vi "Live_Spectrum.vi"() -> ()   [LabVIEW 2022 SP3]
uses:
  PreferencesControl.ctl
  Mic/Mic_Global.vi
  <vilib>/sound2/lvsound2.llb/Sound Input Read (DBL).vi
panel:
  in  "Mode":enum16{"Single Shot", "Continuous"}(ring)
  out "Hammer FFT":cluster{"x0":dbl, "df":dbl, dbl[]}(graph)
  out "Microphone FFT":cluster{"x0":dbl, "df":dbl, dbl[]}(graph)
  in  "Fire":bool
  out "Hammer":waveform(dbl)(graph)
  out "Microphone":waveform(dbl)(graph)
  out "Settings":T1={"Name of test"="", "Date"=timestamp(0 s since 1904-01-01), "Location"="", "Template"="", "Soundcard"="", "resolution"=32, "Sampling rate"=48000, "Ch1 Gain "=25.0, "Ch2 Gain"=10.0, "Sample time (s)"=0.3, "Pre-trigger (s)"=0.01, "Hammer Threshold"=10.0, "Positions"=12, "Taps/Position"=5, "Set Names"="", "Freq resolution"=10.0, "Hammer cutoff"=0.0, "Mic cutoff"=0.0, "Double bounce "=0.0, "Hammer Cal"=10.0, "dB Offset"=0.0, "Accel Cal"=10.0, "Vibrometer Cal"=0.0, "Mic Cal"=1.0, "Output"=2, "Voltage Cal"=1.0, "Vibrometer Port"="ASRL27::INSTR", "Range"=4, "High Pass"=2, "Bandwidth"=4, "X Range"=[], "Y Range"=[], "dB Spread"=0.0, "Trigger"=0, "Ch_1"=25, "Ch_2"=25, "flip?"=FALSE, "60Hz"=FALSE, "Time offset"=0.0, "Piezo Cal"=1.0, "Default Notes"=""} {"Ch_2" min=1 step=1; "Ch_1" min=1 max=100 step=1; "Trigger" items=["Hammer (force)", "Self-tap", "Spacebar"]; "Bandwidth" items=["1 kHz"=1, "5 kHz"=5, "10 kHz"=10, "25 kHz"=25, "50 kHz"=50, "100 kHz"=100]; "High Pass" items=["Off", "13 Hz", "104 Hz"]; "Range" items=["10 mm/s"=1, "20 mm/s"=2, "50 mm/s"=5, "100 mm/s"=10, "200 mm/s"=20, "500 mm/s"=50, "1 m/s"=100, "2 m/s"=200]; "Output" items=["Accelerometer", "Speed (from acceleration)", "Microphone", "Vibrometer", "Piezo"]; "Voltage Cal" format="%#_13g"; "Ch2 Gain" format="%#_13g"; "Ch1 Gain" format="%#_13g"; "Double bounce" min=0.0; "Mic cutoff" min=0.0 format="%#_4g"; "Hammer cutoff" min=0.0 format="%#_4g"; "Freq resolution" min=0.0; "Pre-trigger (s)" format="%#_13g"; "Date" format="%<%H:%M\n%d/%m/%y>T"; "resolution" items=["16 bit"=16, "24 bit"=24, "32 bit"=32]; "Sampling rate" items=["22050 samp/s"=22050, "44100 samp/s"=44100, "48000 samp/s"=48000]}
  # "Hz"
  # "dB"
  # "dB"
  # "sec"
  # "sec"
  # "mV/Pa"
  # "mV/m/s2"
  # "mV/mm/s"
  # "V/N"
  # "sec"
  # "sec"
  # "mV/N"
  # "a.u."
  # "a.u."
  # "sec"
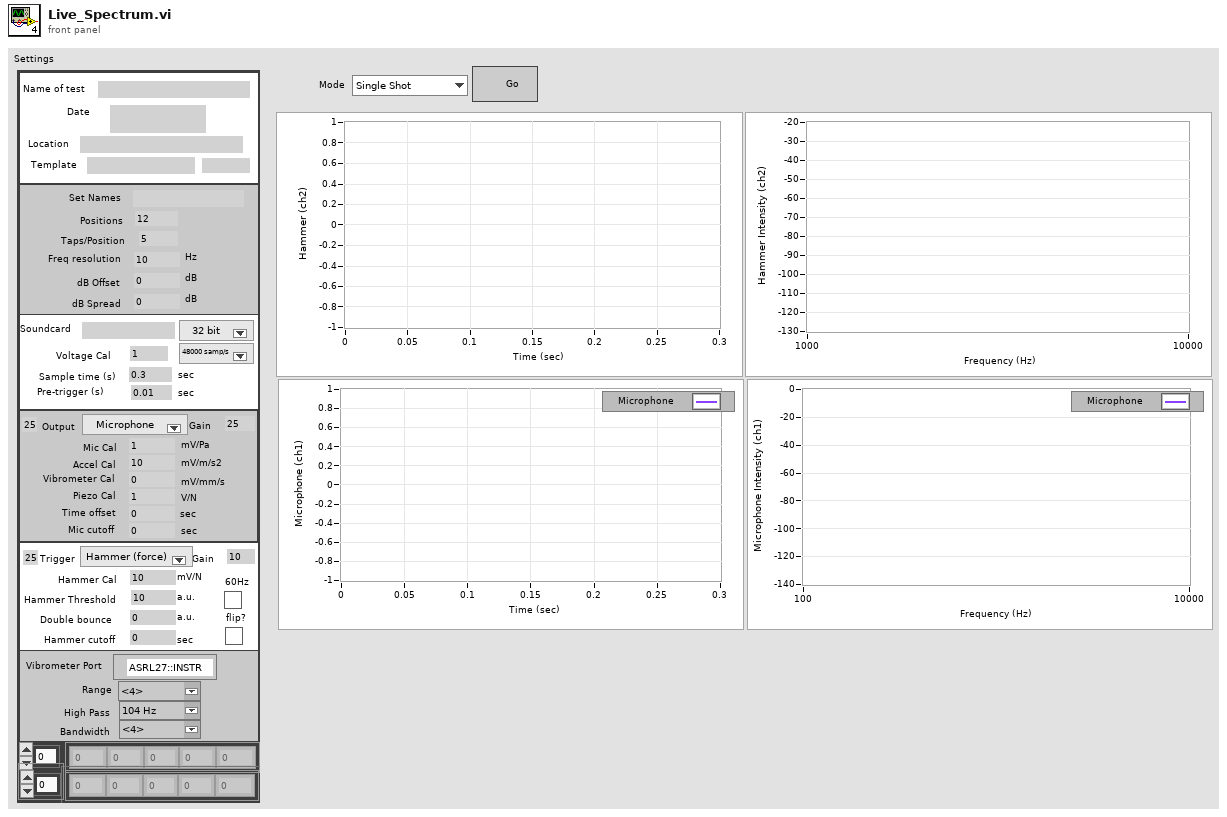
[diagram p1: front panel]
types:
  T1 = typedef "PreferencesControl.ctl" = cluster{"Name of test":string, "Date":timestamp, "Location":string, "Template":string, "Soundcard":string, "resolution":u16, "Sampling rate":u16, "Ch1 Gain ":dbl, "Ch2 Gain":dbl, "Sample time (s)":dbl, "Pre-trigger (s)":dbl, "Hammer Threshold":dbl, "Positions":i16, "Taps/Position":i16, "Set Names":string, "Freq resolution":dbl, "Hammer cutoff":dbl, "Mic cutoff":dbl, "Double bounce ":dbl, "Hammer Cal":dbl, "dB Offset":dbl, "Accel Cal":dbl, "Vibrometer Cal":dbl, "Mic Cal":dbl, "Output":u16, "Voltage Cal":dbl, "Vibrometer Port":refnum<visa-resource-name>, "Range":u16, "High Pass":u16, "Bandwidth":u16, "X Range":cluster{"Minimum":dbl, "Maximum":dbl, "Increment":dbl, "Minor Increment":dbl, "Start":dbl}[], "Y Range":cluster{"Minimum":dbl, "Maximum":dbl, "Increment":dbl, "Minor Increment":dbl, "Start":dbl}[], "dB Spread":dbl, "Trigger":u16, "Ch_1":u8, "Ch_2":u8, "flip?":bool, "60Hz":bool, "Time offset":dbl, "Piezo Cal":dbl, "Default Notes":string}
  T2 = typedef "Sound Input Task ID.ctl" = u32
  T3 = cluster{"task ID":T2, "Num Pts":i32, "timeout":dbl, "FIFO":i32, "Double Bounce":dbl}
  T4 = cluster{"Alerts":bool, "Log X Axis":bool, "dB scale":bool, "Averaging":bool, "Fade":dbl, "Centroids?":bool}
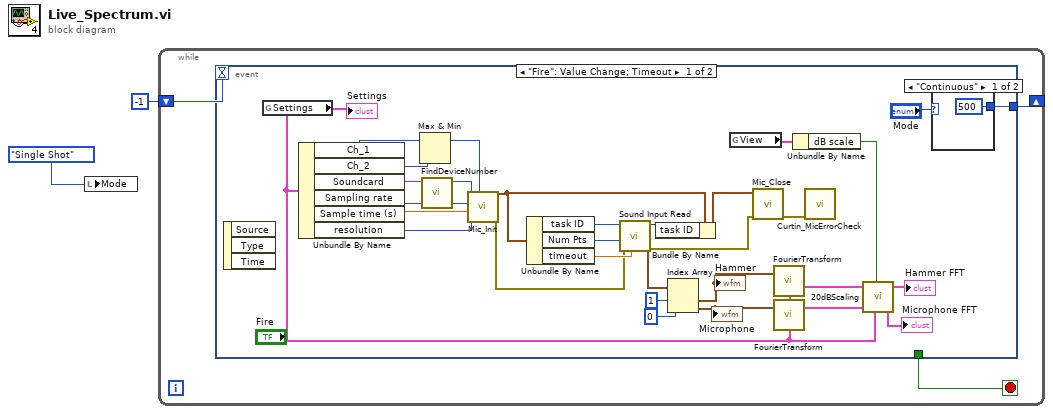
[diagram p0: block diagram]
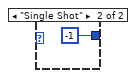
[diagram p2: hidden frame]
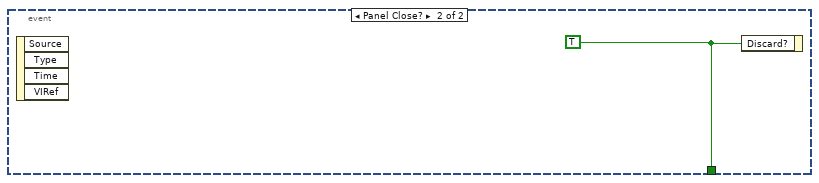
[diagram p3: hidden frame]
diagram:
  n1 = local write "Mode"(enum16{"Single Shot", "Continuous", "Triggered"}."Single Shot" ("Mode")) -> ()
  n2 = while {
    shift-right: [w3] -> _
    shift-left: -1 -> [w4]
    stop <- w5 stop-if-true
    n3 = event shown="[0] \"Fire\": Value Change;  Timeout" {
      selector: _ -> [_ _]
      dyn-events: _ -> [_ _]
      timeout: w4 -> [_ _]
      tunnel: [_ w39] -> w5
      tunnel: [w9 _] -> w3
      event "Fire": Value Change; Timeout {
        n4 = event-data() -> ()  [unwired: 1 in, 3 out]
        n5 = global read "Mic_Global.vi" "Settings"() -> (w15:T1)
        "Settings" <- w15
        n6 = Unbundle By Name(w15) -> ("Ch_1"=w8:u8, "Ch_2"=w7:u8, "Soundcard"=w36:string, "Sampling rate"=w34:u16, "Sample time (s)"=w33:dbl, "resolution"=w32:u16)
        n7 = Max & Min(x=w8, y=w7) -> (max(x,y)=w6:u8)  [unwired: 1 out]
        n8 = call "FindDeviceNumber.vi"("device"=w36) -> ("device"=w35:u16)  [unwired: 10 in]
        n9 = call "Mic_Init.vi"("# channels"=w6, "resolution"=w32, "Sample time"=w33, "Sampling rate"=w34, "device"=w35) -> ("error out"=w25:errorcluster, "DAQ Prams"=w27:T3)  [unwired: 5 in]
        n10 = Unbundle By Name(w27) -> ("task ID"=w31:T2, "Num Pts"=w30:i32, "timeout"=w29:dbl)
        n11 = call-poly <vilib>:"Sound Input Read.vi"("timeout (sec)"=w29, "number of samples/ch"=w30, "error in (no error)"=w25, "task ID"=w31) -> ("error out"=w23:errorcluster, "data"=w24:waveform(dbl)[], "task ID out"=w28:T2)  [unwired: 5 in]
        n12 = Bundle By Name(cluster=w27, "task ID"=w28) -> (w26:T3)
        n13 = Index Array(array=w24, index #1=1 ("index"), index #2=0 ("index")) -> (element #1=w21:waveform(dbl), element #2=w20:waveform(dbl))
        "Hammer" <- w21
        "Microphone" <- w20
        n14 = global read "Mic_Global.vi" "View"() -> (w17:T4)
        n15 = call "Mic_Close.vi"("error in (no error)"=w23, "DAQ Prams"=w26) -> ("error out"=w22:errorcluster)  [unwired: 9 in]
        n16 = call "FourierTransform.vi"("Settings"=w15, "Data"=w21) -> ("FFT"=w14:cluster{dbl, "df":dbl, "FFT {X}":cdb[]})  [unwired: 2 in, 1 out]
        n17 = call "FourierTransform.vi"("Settings"=w15, "Data"=w20) -> ("FFT"=w13:cluster{dbl, "df":dbl, "FFT {X}":cdb[]})  [unwired: 2 in, 1 out]
        n18 = Unbundle By Name(w17) -> ("dB scale"=w16:bool)
        n19 = call "Curtin_MicErrorCheck.vi"("error in (no error)"=w22) -> ()  [unwired: 11 in]
        n20 = call "20dBScaling.vi"("Average FRF in"=w14, "dB?"=w16, "Coherence in"=w13, "Settings"=w15) -> ("Average FRF out"=→"Hammer FFT":cluster{"x0":dbl, "df":dbl, dbl[]}, "Coherence out"=→"Microphone FFT":cluster{"x0":dbl, "df":dbl, dbl[]})  [unwired: 2 in]
        n21 = case shown="\"Continuous\"" "Mode" {
          tunnel: [500 -1] -> w9
          frame "Continuous" {
          }
          frame "Single Shot" {
          }
        }
      }
      event Panel Close? {
        w39 = TRUE ("Discard?")
        n22 = event-data() -> ()  [unwired: 1 in, 4 out]
        n23 = event-data("Discard?"=w39) -> ()  [unwired: 1 in, 1 out]
      }
    }
  }
